vi "Convert Crate Drawing to IDs.vi"(1 "Crate Drawing":string) -> (0 "Crate IDs":string)   [LabVIEW 2020, in "AoC 2022.lvlib"]
uses:
  AoC 2022.lvlib
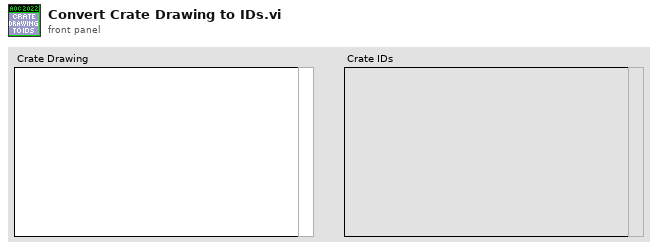
[diagram p1: front panel]
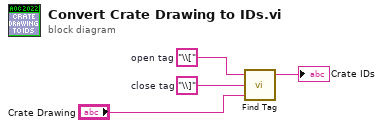
[diagram p0: block diagram]
diagram:
  w3 = "\\]"  # close tag
  w2 = "\\["  # open tag
  n1 = call <vilib>:"Find Tag.vi"("string"="Crate Drawing", "close tag"=w3, "open tag"=w2) -> ("string out"=→"Crate IDs":string)  [unwired: 2 out]
